vi "UTIL_Send Open to Error Queue v1_0_0.vi"(7 "Append file? (False)":bool=TRUE, 8 "error in (no error)":errorcluster, 11 "name (Error)":string="Error") -> (0 "error out":errorcluster)   [LabVIEW 2015]
doc: "UTIL_Send Open to Error Queue v1_0_0.vi\n\nThis vi Sends an open command to the Error Q.vi. It will cause the Error Q.vi to put a note in the error log with a current time stamp stating that the error logging was started.\n\nNote: if the Error Q.vi is not running this will prompt the user with an error.\n\nCreated 2006 by\n\nJ. Daren Suntych\nNational Analytics\n970-397-0764"
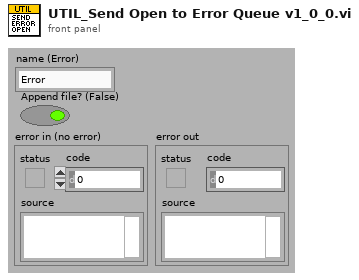
[diagram p1: front panel]
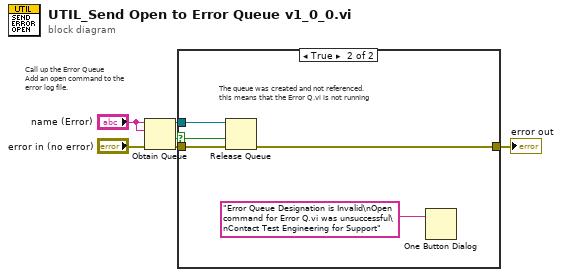
[diagram p0: block diagram]
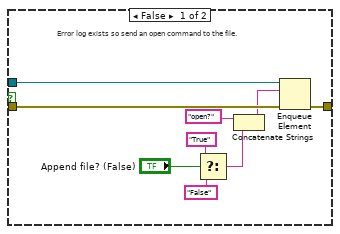
[diagram p2: hidden frame]
diagram:
  # "Call up the Error Queue\nAdd an open command to the \nerror log file."
  n1 = Obtain Queue(name (unnamed)="name (Error)", element data type="name (Error)", error in (no error)="error in (no error)") -> (queue out=w4:refnum<queue>, created new?=w2:bool, error out=w3:errorcluster)  [unwired: 2 in]
  n2 = case shown="True" w2 {
    selector: w2 -> [_ w18]
    tunnel: w4 -> [w15 w20]
    tunnel: w3 -> [w14 w19]
    tunnel: [w13 w17] -> w1
    frame False {
      # "Error log exists so send an open command to the file."
      n3 = Select(t="True" ("queue element"), s="Append file? (False)", f="False" ("queue element")) -> (s? t:f=w12:string)
      n4 = Concatenate Strings("open?" ("queue element"), w12) -> (w7:string)
      n5 = Enqueue Element(queue=w15, element=w7, error in (no error)=w14) -> (error out=w13:errorcluster)  [unwired: 3 out]
    }
    frame True {
      # "The queue was created and not referenced.  \nthis means that the Error Q.vi is not running"
      n6 = Release Queue(queue=w20, force destroy? (F)=w18, error in (no error)=w19) -> (error out=w17:errorcluster)  [unwired: 2 out]
      n7 = One Button Dialog(message="Error Queue Designation is Invalid\nOpen command for Error Q.vi was unsuccessful\nContact Test Engineering for Support" ("window title (\"\")")) -> ()  [unwired: 2 out]
    }
  }
  "error out" <- w1
